vi "ValveParameters.vi"() -> ()   [LabVIEW 2012]
panel:
  in  "ValveParameters":T1={"baudrate"=9600, "databits"=8, "paritybit"=0, "stopbits"=1, "flux control"=0, "Port"="COM2", "Serial Parameters"={"Mode"=enum."RTU", "Slave Address"=1}, "Timeout"=0, "Valve mapping"={"Inlet Valve"=0, "V1"=1, "V2"=2, "Sample Valve"=3, "Outlet Valve"=4}}
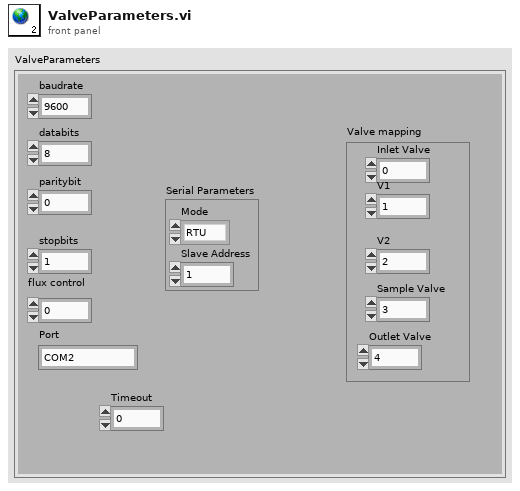
[diagram p1: front panel]
types:
  T1 = cluster{"baudrate":u32, "databits":u16, "paritybit":u16, "stopbits":u16, "flux control":u16, "Port":string, "Serial Parameters":cluster{"Mode":enum16{"RTU", "ASCII"}, "Slave Address":u8}, "Timeout":u32, "Valve mapping":cluster{"Inlet Valve":u8, "V1":u8, "V2":u8, "Sample Valve":u8, "Outlet Valve":u8}}
diagram:
